vi "get initial information.vi"(8 "error in (no error)":errorcluster, 10 "channel":u16, 11 "Simulated_CCD_Camera in":refnum<class "Sim_Ixon_Ultra.lvclass">) -> (0 "error out":errorcluster, 2 "ccd on/off":bool, 3 "Simulated_CCD_Camera out":refnum<class "Sim_Ixon_Ultra.lvclass">)   [LabVIEW 2018, in "Sim_Ixon_Ultra.lvclass"]
uses:
  Sim_Ixon_Ultra.lvclass
  Sim_Ixon_Ultra.lvclass/Sim_Ixon_Ultra.ctl
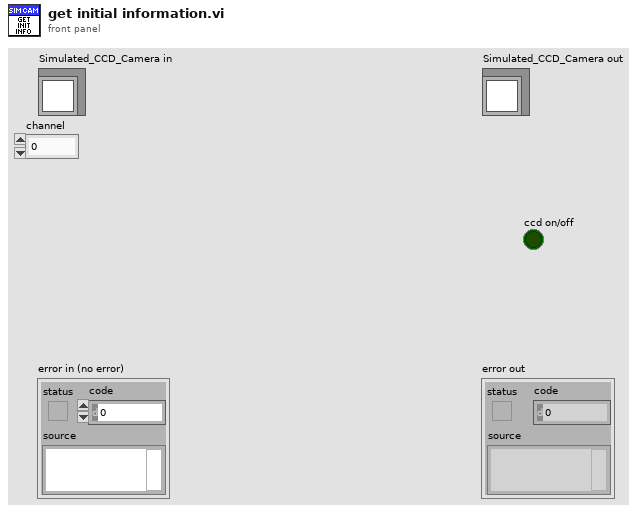
[diagram p1: front panel]
types:
  T1 = cluster{"CYCLES_DONE":u16, "LAST_IMAGE_NAME":string, "USED_DISK_SPACE":u16, "FRAMES_DONE":u16, "CCD_STATUS":string, "CURRENT_TEMPERATURE":i16, "TEMPERATURE_STATUS":string, "FRAME_EXPOSURE_TIME":sgl, "ERROR":bool, "SERIAL_NUMBER":u16, "ACQUIRING":bool, "IMAGE_INDEX":u32, "SEQS_DONE":u16}
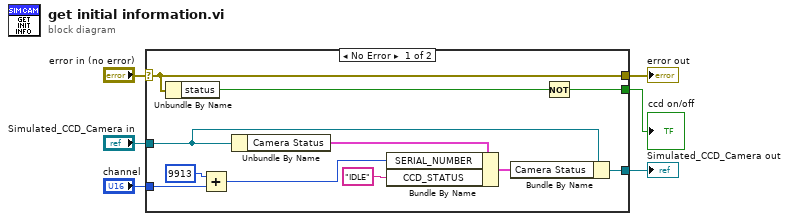
[diagram p0: block diagram]
diagram:
  n1 = case shown="No Error" "error in (no error)" {
    selector: "error in (no error)" -> [w10 w19]
    tunnel: [w10 w19] -> w4
    tunnel: [w16 w18] -> w3
    tunnel: "Simulated_CCD_Camera in" -> [w15 w18]
    tunnel: "channel" -> [w13 _]
    tunnel: [w8 _] -> w1
    frame No Error {
      n2 = Unbundle By Name(w10) -> ("status"=w9:bool)
      n3 = Add(x=u16 9913 ("Initialization.Serial Number"), y=w13) -> (x+y=w7:u16)
      n4 = Unbundle By Name(w15) -> ("Camera Status"=w12:T1)
      n5 = Bundle By Name(cluster=w12, "SERIAL_NUMBER"=w7, "CCD_STATUS"="IDLE" ("Camera Status.STATUS")) -> (w11:T1)
      n6 = Bundle By Name(cluster=w15, "Camera Status"=w11) -> (w16:refnum<class "Sim_Ixon_Ultra.lvclass">)
      n7 = Not(x=w9) -> (.not. x?=w8:bool)
    }
    frame Error {
    }
  }
  "error out" <- w4
  "Simulated_CCD_Camera out" <- w3
  "ccd on/off" <- w1
